vi "AdvFilter-Enumerate Valid Params.vi"(8 "error in (no error)":errorcluster, 11 "Filter":T1(xcontrol)) -> (0 "error out":errorcluster, 2 "Parameter Names":string[](array[string]))   [LabVIEW 2015]
uses:
  Controls/Filter XCtl/Filter XCtl.xctl
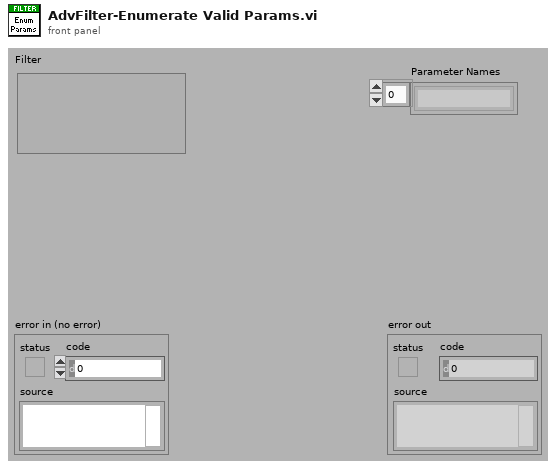
[diagram p1: front panel]
types:
  T1 = cluster{"CF (kHz)":dbl, "BW (kHz)":dbl, "IIR Filter Cluster":cluster{"filter structure":enum32{"IIR 2nd Order", "IIR 4th Order"}, "Reverse Coefficients":dbl[], "Forward Coefficients":dbl[]}, "Final Filter State":dbl[], "Scale Factor":dbl, "Final Filter State 2":dbl[], "Quadrature":bool, "Type":enum16{"Lowpass", "Highpass", "Bandpass", "Bandstop", "OFF"}}
  T2 = enum16{"Lowpass", "Highpass", "Bandpass", "Bandstop", "OFF"}
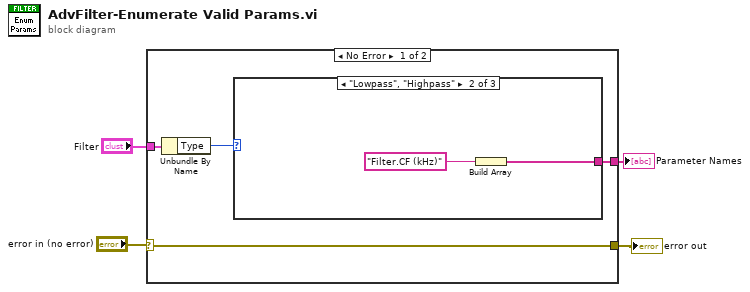
[diagram p0: block diagram]
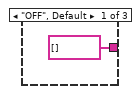
[diagram p2: hidden frame]
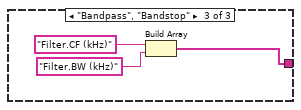
[diagram p3: hidden frame]
diagram:
  n1 = case shown="No Error" "error in (no error)" {
    selector: "error in (no error)" -> [w5 w15]
    tunnel: "Filter" -> [w7 _]
    tunnel: [w6 _] -> w3
    tunnel: [w5 w15] -> w1
    frame No Error {
      n2 = Unbundle By Name(w7) -> ("Type"=w8:T2)
      n3 = case shown="\"Lowpass\", \"Highpass\"" w8 {
        tunnel: [string[] [] w10 w12] -> w6
        frame "OFF", Default {
        }
        frame "Lowpass", "Highpass" {
          n4 = Build Array("Filter.CF (kHz)" ("String")) -> (w10:string[])
        }
        frame "Bandpass", "Bandstop" {
          n5 = Build Array("Filter.CF (kHz)" ("String"), "Filter.BW (kHz)" ("String")) -> (w12:string[])
        }
      }
    }
    frame Error {
    }
  }
  "error out" <- w1
  "Parameter Names" <- w3
